vi "transformed1.vi"() -> ()   [LabVIEW 2018]
uses:
  subs/path list.vi
  <vilib>/Analysis/NI_AALPro.lvlib
  <vilib>/Analysis/NI_AALBase.lvlib
panel:
  out "?":dbl[](graph)
  in  "transformed":dbl format="%.2f"
  out "B":dbl=22.2 format="%.2f"
  in  "multiply factor":dbl=1000000.0 format="%.2e"
  in  "n norm":u8=5
  in  "# interp":dbl=1023.0 format="%.2f"
  in  "# points":u32=101
  in  "B max":dbl=32.0 format="%.4f"
  in  "B min":dbl=22.0 format="%.4f"
  in  "save plots?":bool=TRUE
  in  "format":string="%.6e"
  in  "temperatures":dbl[](array[numeric]) format="%.4f"
  out "plotted data":cluster{dbl[], dbl[]}[](graph)
  in  "type of interpolation":u16(ring) items=["linear", "cubic spline", "polynomial"]
  in  "y domain":u16(ring) items=["channel A"]
  in  "x domain":u16(ring) items=["B (rising field)", "B (falling field)"]
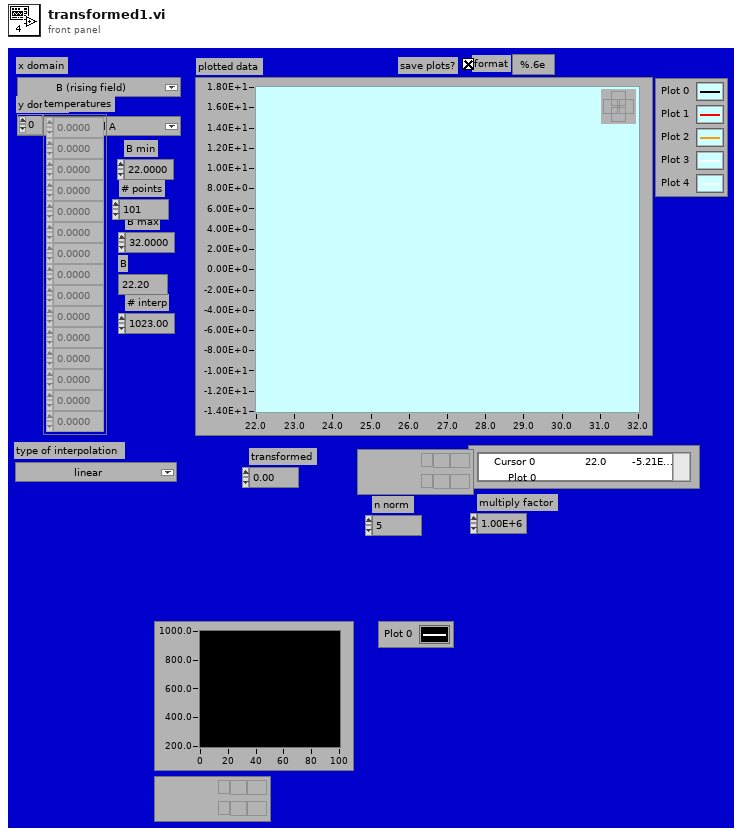
[diagram p1: front panel]
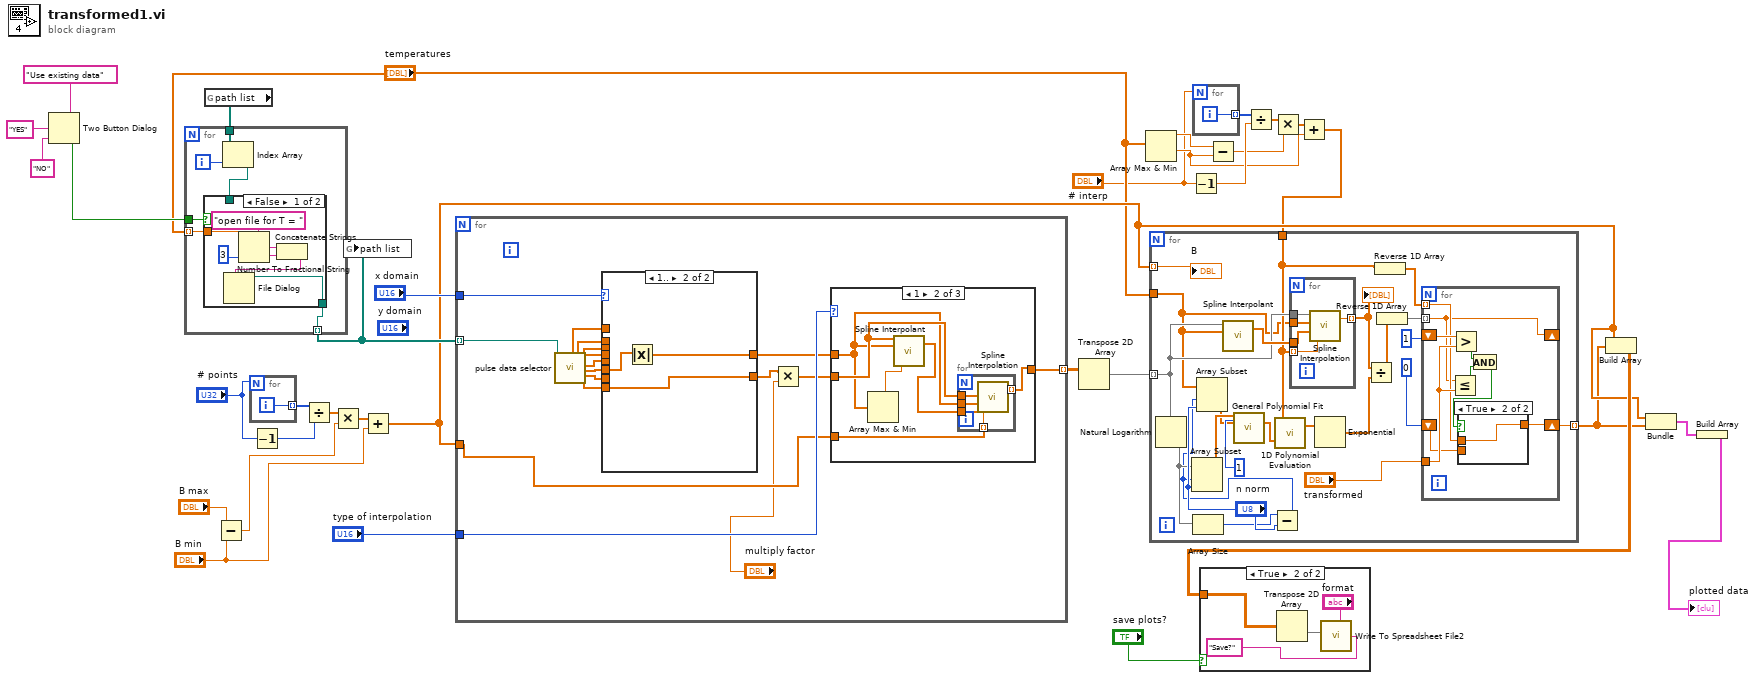
[diagram p0: block diagram]
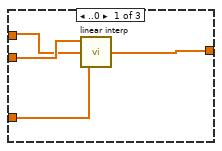
[diagram p5: hidden frame]
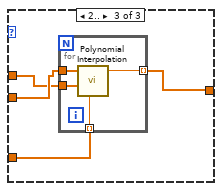
[diagram p6: hidden frame]
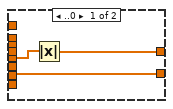
[diagram p7: hidden frame]
diagram:
  n1 = Two Button Dialog(message="Use existing data", 1:"NO", 2:"YES") -> (T button?=w27:bool)
  n2 = global read "path list.vi" "path list"() -> (w31:path[])
  n3 = for {
    tunnel: "temperatures" -> [w40] mode=indexing
    tunnel: [w39] -> w32 mode=indexing
    tunnel: w31 -> [w37]
    tunnel: w27 -> [w38]
    i -> [w36]
    n4 = Index Array(array=w37, index=w36) -> (element=w35:path)
    n5 = case shown="False" w38 {
      tunnel: w40 -> [w42 _]
      tunnel: [w41 w47] -> w39
      tunnel: w35 -> [_ w47]
      frame False {
        n6 = Number To Fractional String(number=w42, precision (6)=3) -> (F-format string=w45:string)  [unwired: 2 in]
        n7 = Concatenate Strings("open file for T = ", w45) -> (w46:string)
        n8 = File Dialog(7:w46) -> (3:w41:path)  [unwired: 6 in, 3 out]
      }
      frame True {
      }
    }
  }
  n9 = Subtract(x="B max", y="B min") -> (x-y=w22:dbl)
  n10 = for {
    N: "# points" -> [_]
    tunnel: [w48] -> w24 mode=indexing
    i -> [w48]
  }
  n11 = Decrement(x="# points") -> (x-1=w25:u32)
  n12 = Divide(x=w24, y=w25) -> (x/y=w21:dbl[])
  n13 = Multiply(x=w21, y=w22) -> (x*y=w20:dbl[])
  n14 = global write "path list.vi" "path list"(w32) -> ()
  n15 = Add(x=w20, y="B min") -> (x+y=w15:dbl[])
  n16 = for {
    tunnel: "x domain" -> [w57]
    tunnel: "type of interpolation" -> [w55]
    tunnel: w32 -> [w56] mode=indexing
    tunnel: w15 -> [w53]
    tunnel: [w52] -> w18 mode=indexing
    n17 = call "pulse data selector.vi"("file path (dialog if empty)"=w56) -> ("time rising"=w60:dbl[], "time falling"=w61:dbl[], "dB/dt rising"=w59:dbl[], "dB/dt falling"=w58:dbl[], "B rising"=w64:dbl[], "B falling"=w65:dbl[], "ch A rising"=w62:dbl[], "ch A falling"=w63:dbl[])  [unwired: 6 in, 5 out]
    n18 = case shown="1.." w57 {
      tunnel: w60 -> [_ _]
      tunnel: w61 -> [_ _]
      tunnel: w62 -> [w90 _]
      tunnel: w63 -> [_ w92]
      tunnel: w64 -> [w91 _]
      tunnel: w65 -> [_ w94]
      tunnel: w59 -> [_ _]
      tunnel: w58 -> [_ _]
      tunnel: [w90 w92] -> w51
      tunnel: [w89 w93] -> w54
      frame ..0 {
        n19 = Absolute Value(x=w91) -> (abs(x)=w89:dbl[])
      }
      frame 1.. {
        n20 = Absolute Value(x=w94) -> (abs(x)=w93:dbl[])
      }
    }
    n21 = Multiply(x=w51, y="multiply factor") -> (x*y=w50:dbl[])
    n22 = case shown="1" w55 {
      tunnel: w54 -> [w68 w72 w83]
      tunnel: w50 -> [w69 w73 w84]
      tunnel: [w66 w70 w81] -> w52
      tunnel: w53 -> [w67 w74 w82]
      frame ..0 {
        n23 = call "linear interp.vi"("x array"=w67, "X data"=w68, "Y data"=w69) -> ("y"=w66:dbl[])
      }
      frame 1 {
        n24 = Array Max & Min(array=w72) -> (max value=w75:dbl)  [unwired: 3 out]
        n25 = call <vilib>:"Spline Interpolant.vi"("final boundary"=w75, "X"=w72, "Y"=w73) -> ("Interpolant"=w71:dbl[])  [unwired: 1 in, 1 out]
        n26 = for {
          tunnel: w74 -> [w80] mode=indexing
          tunnel: w73 -> [w79]
          tunnel: w72 -> [w78]
          tunnel: w71 -> [w77]
          tunnel: [w76] -> w70 mode=indexing
          n27 = call <vilib>:"Spline Interpolation.vi"("x value"=w80, "Interpolant"=w77, "X"=w78, "Y"=w79) -> ("interpolation value"=w76:dbl)  [unwired: 1 out]
        }
      }
      frame 2.. {
        n28 = for {
          tunnel: w84 -> [w88]
          tunnel: w83 -> [w87]
          tunnel: w82 -> [w86] mode=indexing
          tunnel: [w85] -> w81 mode=indexing
          n29 = call <vilib>:"Polynomial Interpolation.vi"("x value"=w86, "X"=w87, "Y"=w88) -> ("interpolation value"=w85:dbl)  [unwired: 2 out]
        }
      }
    }
  }
  n30 = Transpose 2D Array(2D array=w18) -> (transposed array=w17:dbl[][])
  n31 = Array Max & Min(array="temperatures") -> (max value=w10:dbl, min value=w6:dbl)  [unwired: 2 out]
  n32 = Decrement(x="# interp") -> (x-1=w11:dbl)
  n33 = for {
    N: "# interp" -> [_]
    tunnel: [w95] -> w12 mode=indexing
    i -> [w95]
  }
  n34 = Subtract(x=w10, y=w6) -> (x-y=w9:dbl)
  n35 = Divide(x=w12, y=w11) -> (x/y=w8:dbl[])
  n36 = Multiply(x=w8, y=w9) -> (x*y=w7:dbl[])
  n37 = Add(x=w7, y=w6) -> (x+y=w5:dbl[])
  n38 = for {
    tunnel: w15 -> [w118] mode=indexing
    tunnel: "temperatures" -> [w107]
    tunnel: w17 -> [w116] mode=indexing
    tunnel: w5 -> [w111]
    tunnel: [w98] -> w4 mode=indexing
    n39 = Natural Logarithm(1:w116) -> (0:w105:dbl[])
    n40 = Array Size(array=w105) -> (size(s)=w104:i32)
    n41 = call <vilib>:"Spline Interpolant.vi"("X"=w107, "Y"=w116) -> ("Interpolant"=w117:dbl[])  [unwired: 2 in, 1 out]
    n42 = Subtract(x=w104, y="n norm") -> (x-y=w103:i32)
    n43 = Array Subset(array=w105, index=w103, length="n norm") -> (w102:dbl[])
    n44 = Array Subset(array=w107, index=w103, length="n norm") -> (w101:dbl[])
    n45 = call <vilib>:"General Polynomial Fit.vi"("Y"=w102, "polynomial order"=1, "X"=w101) -> ("Polynomial Coefficients"=w114:dbl[])  [unwired: 9 in, 3 out]
    n46 = call <vilib>:"1D Polynomial Evaluation.vi"("Coefficients: a"=w114, "X"=w111) -> ("Y"=w113:dbl[])  [unwired: 1 out]
    n47 = for {
      tunnel: w116 -> [w134]
      tunnel: w107 -> [w133]
      tunnel: w117 -> [w132]
      tunnel: w111 -> [w131] mode=indexing
      tunnel: [w130] -> w97 mode=indexing
      n48 = call <vilib>:"Spline Interpolation.vi"("x value"=w131, "Interpolant"=w132, "X"=w133, "Y"=w134) -> ("interpolation value"=w130:dbl)  [unwired: 1 out]
    }
    "?" <- w97
    n49 = Exponential(1:w113) -> (0:w112:dbl[])
    n50 = Divide(x=w97, y=w112) -> (x/y=w96:dbl[])
    n51 = Reverse 1D Array(array=w111) -> (reversed array=w110:dbl[])
    n52 = Reverse 1D Array(array=w96) -> (reversed array=w109:dbl[])
    n53 = for {
      tunnel: w110 -> [w123] mode=indexing
      tunnel: w109 -> [w120] mode=indexing
      shift-right: [w120] -> _
      shift-left: 1 -> [w127]
      tunnel: "transformed" -> [w126]
      shift-right: [w121] -> w98
      shift-left: 0 -> [w122]
      n54 = Less Or Equal?(x=w120, y=w126) -> (x <= y?=w124:bool)
      n55 = Greater?(x=w127, y=w126) -> (0:w125:bool)
      n56 = And(x=w125, y=w124) -> (x .and. y?=w119:bool)
      n57 = case shown="True" w119 {
        tunnel: w123 -> [_ w129]
        tunnel: w122 -> [w128 _]
        tunnel: [w128 w129] -> w121
        frame False {
        }
        frame True {
        }
      }
    }
    "B" <- w118
  }
  n58 = Build Array(w15, w4) -> (w16:dbl[][])
  n59 = case shown="True" "save plots?" {
    tunnel: w16 -> [_ w135]
    frame False {
    }
    frame True {
      n60 = Transpose 2D Array(2D array=w135) -> (transposed array=w137:dbl[][])
      n61 = call "Write To Spreadsheet File2.vi"("dialogue"="Save?", "format (%.3f)"="format", "2D data"=w137) -> ()  [unwired: 5 in, 1 out]
    }
  }
  n62 = Bundle(w15, w4) -> (w14:cluster{dbl[], dbl[]})  [unwired: 1 in]
  n63 = Build Array(w14) -> (→"plotted data":cluster{dbl[], dbl[]}[])
